vi "Create Chassis BOM.vi"(7 "ChassisType":T1, 8 "error in (no error)":errorcluster, 9 "System Hardware":refnum<k20>, 10 "IP Addr":string, 11 "SysAPI Session":refnum<k21>) -> (0 "error out":errorcluster, 2 "Chassis BOM out":refnum<class "Chassis BOM.lvclass">, 3 "SysAPI Session":refnum<k21>, 5 "Chassis Meta Data":string[](array[string]))   [LabVIEW 2012, in "Configuration Grandmaster.lvlib" / "Chassis BOM.lvclass"]
uses:
  Chassis BOM.lvclass
  Common/Controls/Chassis Type.ctl
  DAQmx Mod Info.ctl
  Chassis BOM.lvclass/Chassis BOM.ctl
  <vilib>/nisyscfg/Find Hardware.vi
  <resource>/objmgr/nisysapi.rc
  <vilib>/nisyscfg/nisyscfg.lvlib
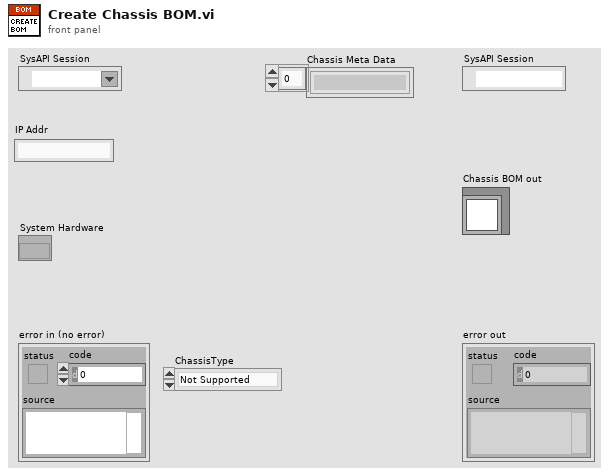
[diagram p1: front panel]
types:
  T1 = typedef "Chassis Type.ctl" = enum16{"Not Supported", "C Series 1-Slot", "C Series 4-Slot", "C Series 8-Slot", "PXI 8-Slot", "PXIe 18-Slot"}
  T2 = typedef "Configuration Grandmaster.lvlib/Chassis BOM.lvclass/DAQmx Mod Info.ctl" = cluster{"Slot Number":i32, "DAQmx Alias":string}
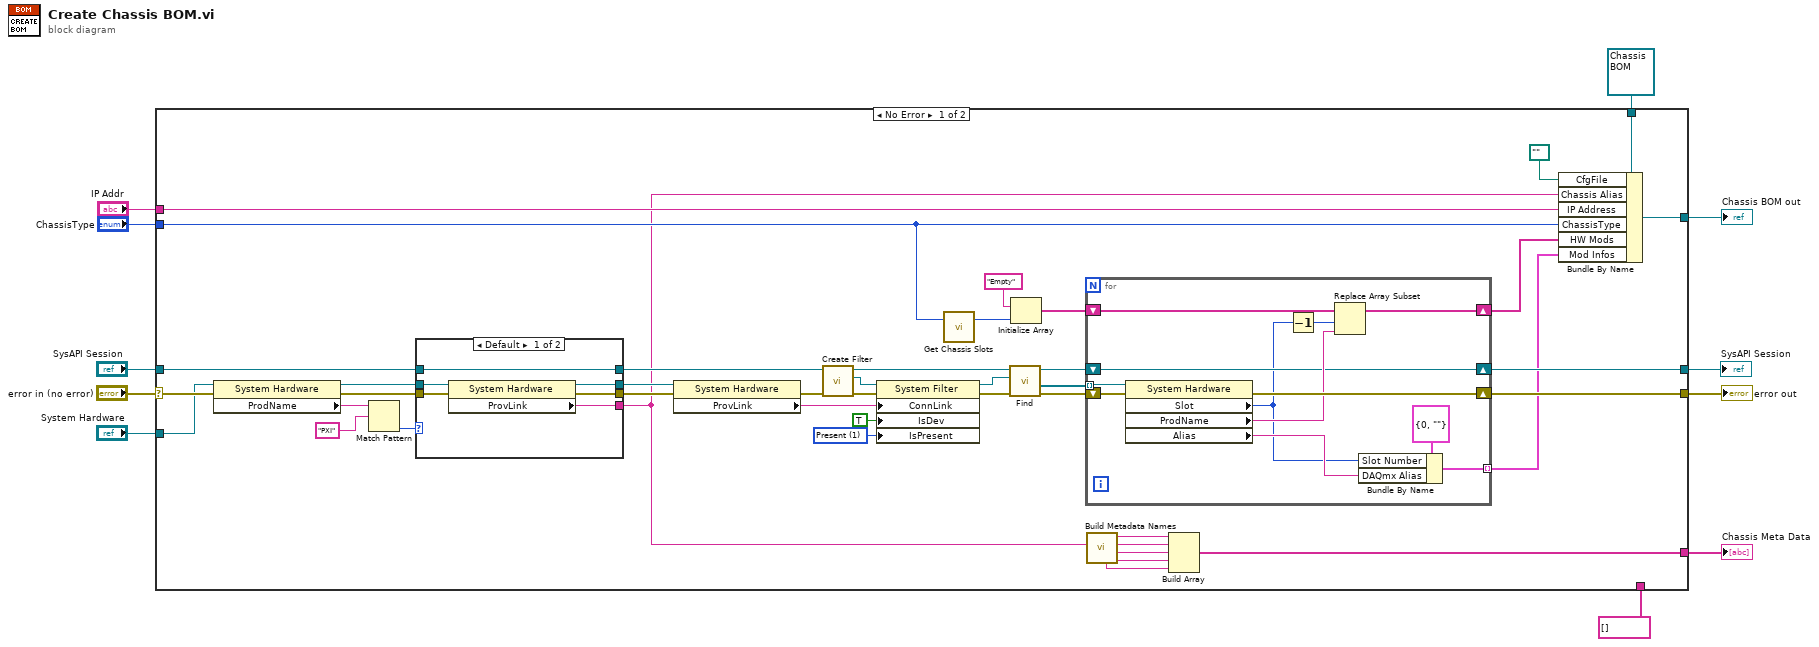
[diagram p0: block diagram]
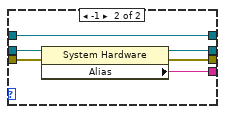
[diagram p2: hidden frame]
diagram:
  n1 = case shown="No Error" "error in (no error)" {
    selector: "error in (no error)" -> [w47 w81]
    tunnel: [w48 w81] -> w10
    tunnel: [w52 w80] -> w8
    tunnel: refnum<class "Chassis BOM.lvclass"> refnum ("Chassis BOM in") -> [w53 w80]
    tunnel: "SysAPI Session" -> [w21 w78]
    tunnel: "ChassisType" -> [w26 _]
    tunnel: "System Hardware" -> [w46 _]
    tunnel: [w31 w79] -> w4
    tunnel: string[] [] -> [_ w79]
    tunnel: "IP Addr" -> [w30 _]
    tunnel: [w28 w78] -> w1
    frame No Error {
      w45 = 1 items=["Unknown"=-1, "Not Present"=0, "Present"=1] ("Devices & Chassis:Is Present")
      n2 = property class="System Hardware"(reference=w46, error in=w47) -> (reference out=w20:refnum<k20>, error out=w19:errorcluster, "ProdName"=w23:string)
      n3 = Match Pattern(string=w23, regular expression="PXI") -> (offset past match=w22:i32)  [unwired: 1 in, 3 out]
      n4 = case shown="Default" w22 {
        tunnel: w21 -> [w57 w63]
        tunnel: w20 -> [w59 w65]
        tunnel: w19 -> [w58 w64]
        tunnel: [w57 w63] -> w13
        tunnel: [w55 w62] -> w16
        tunnel: [w56 w61] -> w17
        tunnel: [w54 w60] -> w12
        frame Default {
          n5 = property class="System Hardware"(reference=w59, error in=w58) -> (reference out=w56:refnum<k20>, error out=w55:errorcluster, "ProvLink"=w54:string)
        }
        frame -1 {
          n6 = property class="System Hardware"(reference=w65, error in=w64) -> (reference out=w61:refnum<k20>, error out=w62:errorcluster, "Alias"=w60:string)
        }
      }
      n7 = property class="System Hardware"(reference=w17, error in=w16) -> (error out=w14:errorcluster, "ProvLink"=w15:string)  [unwired: 1 out]
      n8 = call <vilib>:"Create Filter.vi"("error in (no error)"=w14, "session in"=w13) -> ("error out"=w39:errorcluster, "filter out"=w40:refnum<k20>, "session out"=w41:refnum<k21>)  [unwired: 7 in]
      n9 = property class="System Filter"(reference=w40, error in=w39, "ConnLink"=w15, "IsDev"=TRUE ("Is Device"), "IsPresent"=w45) -> (reference out=w43:refnum<k20>, error out=w42:errorcluster)
      n10 = call "Get Chassis Slots.vi"("ChassisType"=w26) -> ("Num of Slots"=w27:i32)  [unwired: 2 in]
      n11 = call-poly <vilib>:"Find.vi"("error in (no error)"=w42, "filter in"=w43, "session in"=w41) -> ("error out"=w38:errorcluster, "resources out"=w37:refnum<k20>[], "session out"=w29:refnum<k21>)  [unwired: 5 in, 1 out]
      n12 = Initialize Array("Empty" ("ProductType"), w27) -> (w50:string[])
      n13 = for {
        shift-right: [w73] -> w48
        shift-left: w38 -> [w74]
        shift-right: [w76] -> w25
        shift-left: w50 -> [w77]
        tunnel: w37 -> [w71] mode=indexing
        shift-right: [w70] -> w28
        shift-left: w29 -> [w70]
        tunnel: [w66] -> w24 mode=indexing
        n14 = property class="System Hardware"(reference=w71, error in=w74) -> (error out=w73:errorcluster, "Slot"=w67:i32, "ProdName"=w72:string, "Alias"=w68:string)  [unwired: 1 out]
        n15 = Decrement(x=w67) -> (x-1=w75:i32)
        n16 = Replace Array Subset(array=w77, new element=w72, index=w75) -> (w76:string[])
        n17 = Bundle By Name(cluster=T2 {"Slot Number"=0, "DAQmx Alias"=""} ("Mod Info"), "Slot Number"=w67, "DAQmx Alias"=w68) -> (w66:T2)
      }
      n18 = call "Build Metadata Names.vi"("Chassis Name"=w12) -> ("Modbus Wfm Hdr"=w33:string, "Modbus Wfm"=w34:string, "Wfm Hdr"=w35:string, "Wfm"=w36:string, "Down"=w32:string)  [unwired: 6 in]
      n19 = Build Array(w36, w35, w34, w33, w32) -> (w31:string[])
      n20 = Bundle By Name(cluster=w53, "CfgFile"=path "", "Chassis Alias"=w12, "IP Address"=w30, "ChassisType"=w26, "HW Mods"=w25, "Mod Infos"=w24) -> (w52:refnum<class "Chassis BOM.lvclass">)
    }
    frame Error {
    }
  }
  "error out" <- w10
  "Chassis BOM out" <- w8
  "Chassis Meta Data" <- w4
  "SysAPI Session" <- w1
